vi "Query Output On Off.vi"(7 "Slave Address":i32=-1 min=-1 max=30 step=1, 8 "error":errorcluster, 11 "VISA":refnum<visa-resource-name>) -> (0 "error out":errorcluster, 2 "Output ON":bool, 3 "VISA out":refnum<visa-resource-name>)   [LabVIEW 2025, in "TDK-Lambda GEN LAN Series.lvlib"]
doc: "Reads the output state and returns a boolean:\n TRUE if the power supply output is ON and \n FALSE if the power supply output is OFF."
uses:
  <userlib>/TDK-Lambda GEN LAN Series/TDK-Lambda GEN LAN Series.lvlib
panel:
  # "TDK-Lambda Genesys \n LAN\n  DC Power Supplies"
  # "Read:\n Output ON or OFF"
  # "(c) 2019 TDK-Lambda.  ALL RIGHTS RESERVED."
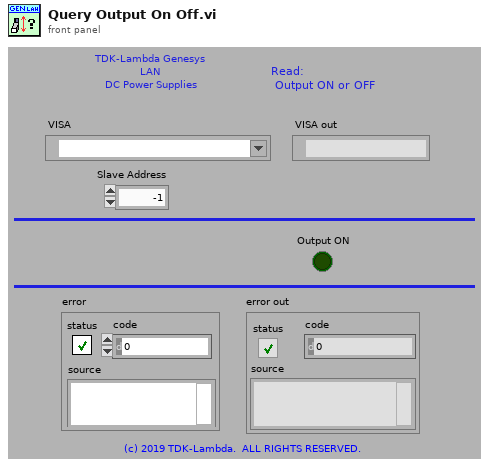
[diagram p1: front panel]
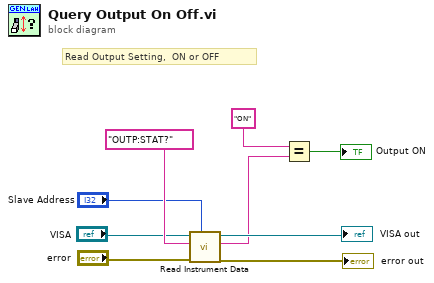
[diagram p0: block diagram]
diagram:
  # "Read Output Setting,  ON or OFF"
  n1 = call <userlib>:"Read Instrument Data.vi"("Slave Address"="Slave Address", "error"="error", "Query"="OUTP:STAT?" ("format string"), "VISA"="VISA") -> ("error out"=→"error out":errorcluster, "Response"=w6:string, "VISA out"=→"VISA out":refnum<visa-resource-name>)  [unwired: 4 in, 1 out]
  n2 = Equal?(x="ON" ("format string"), y=w6) -> (x = y?=→"Output ON":bool)
